vi "Increment Decrement Visibility.vi"(0 "Control in":refnum<vi>, 5 "make compliant?":bool, 11 "error in":errorcluster) -> (4 "Control out":refnum<vi>, 6 "non-compliant?":bool, 15 "error out":errorcluster)   [LabVIEW 2011, in "Align To Connector.lvlib"]
uses:
  Align To Connector.lvlib
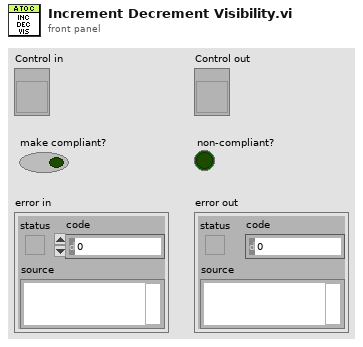
[diagram p1: front panel]
types:
  T1 = enum32{"not a typedef", "typedef", "strict typedef", "class private data"}
  T2 = typedef "LVRectTypeDef.ctl" = cluster{"Left":i16, "Top":i16, "Right":i16, "Bottom":i16}
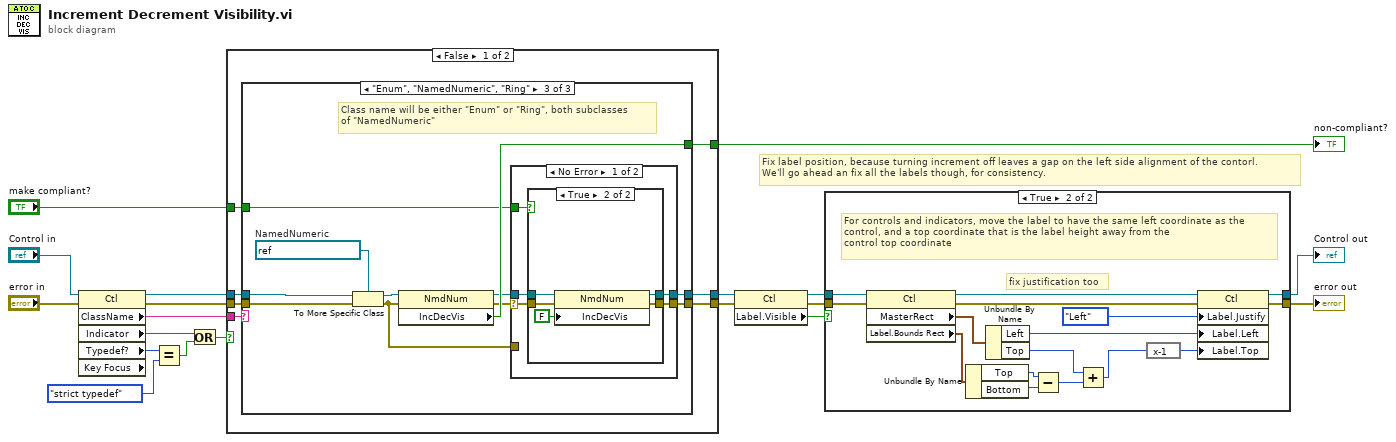
[diagram p0: block diagram]
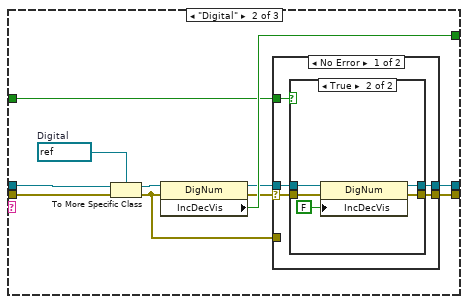
[diagram p4: hidden frame]
diagram:
  # "Fix label position, because turning increment off leaves a gap on the left side alignment of the contorl.\nWe'll go ahead an fix all the labels though, for consistency."
  n1 = property class="Ctl" props=["ClassName", "Indicator", "Typedef?", "Key Focus"](reference="Control in", error in="error in") -> (reference out=w15:refnum<vi>, error out=w14:errorcluster, "ClassName"=w8:string, "Indicator"=w13:bool, "Typedef?"=w12:T1)  [unwired: 1 out]
  n2 = Equal?(x=w12, y=T1."strict typedef" ("x")) -> (x = y?=w10:bool)
  n3 = Or(x=w13, y=w10) -> (x .or. y?=w9:bool)
  n4 = case shown="False" w9 {
    tunnel: [w26 _] -> w19
    tunnel: "make compliant?" -> [w25 _]
    tunnel: [w21 w80] -> w3
    tunnel: [w20 w79] -> w4
    tunnel: w15 -> [w24 w80]
    tunnel: w14 -> [w23 w79]
    tunnel: w8 -> [w22 _]
    frame False {
      n5 = case shown="\"Enum\", \"NamedNumeric\", \"Ring\"" w22 {
        tunnel: [_ w39 w64] -> w26
        tunnel: w25 -> [_ w30 w55]
        tunnel: [w27 w38 w57] -> w21
        tunnel: [w28 w37 w54] -> w20
        tunnel: w23 -> [w28 w34 w62]
        tunnel: w24 -> [w27 w33 w61]
        frame Default {
        }
        frame "Digital" {
          w35 = refnum<vi> refnum  # Digital
          n6 = To More Specific Class(target class=w35, reference=w33, error in=w34) -> (specific class reference=w36:refnum<vi>, error out=w29:errorcluster)
          n7 = property class="DigNum"(reference=w36, error in=w29) -> (reference out=w32:refnum<vi>, error out=w31:errorcluster, "IncDecVis"=w39:bool)
          n8 = case shown="No Error" w31 {
            selector: w31 -> [w41 _]
            tunnel: [w44 w52] -> w38
            tunnel: [w43 w53] -> w37
            tunnel: w32 -> [w42 w52]
            tunnel: w30 -> [w40 _]
            tunnel: w29 -> [_ w53]
            frame No Error {
              n9 = case shown="True" w40 {
                tunnel: [w46 w51] -> w44
                tunnel: [w45 w50] -> w43
                tunnel: w42 -> [w46 w49]
                tunnel: w41 -> [w45 w48]
                frame False {
                }
                frame True {
                  n10 = property class="DigNum"(reference=w49, error in=w48, "IncDecVis"=FALSE ("Increment/Decrement Visible?")) -> (reference out=w51:refnum<vi>, error out=w50:errorcluster)
                }
              }
            }
            frame Error {
              # "clear errors,\nsystem digital ctrls\ndon't have inc/dec"
            }
          }
        }
        frame "Enum", "NamedNumeric", "Ring" {
          w60 = refnum<vi> refnum  # NamedNumeric
          # "Class name will be either \"Enum\" or \"Ring\", both subclasses\nof \"NamedNumeric\""
          n11 = To More Specific Class(target class=w60, reference=w61, error in=w62) -> (specific class reference=w63:refnum<vi>, error out=w56:errorcluster)
          n12 = property class="NmdNum"(reference=w63, error in=w56) -> (reference out=w59:refnum<vi>, error out=w58:errorcluster, "IncDecVis"=w64:bool)
          n13 = case shown="No Error" w58 {
            selector: w58 -> [w66 _]
            tunnel: [w69 w77] -> w57
            tunnel: [w68 w78] -> w54
            tunnel: w59 -> [w67 w77]
            tunnel: w55 -> [w65 _]
            tunnel: w56 -> [_ w78]
            frame No Error {
              n14 = case shown="True" w65 {
                tunnel: [w71 w76] -> w69
                tunnel: [w70 w75] -> w68
                tunnel: w67 -> [w71 w74]
                tunnel: w66 -> [w70 w73]
                frame False {
                }
                frame True {
                  n15 = property class="NmdNum"(reference=w74, error in=w73, "IncDecVis"=FALSE ("Increment/Decrement Visible?")) -> (reference out=w76:refnum<vi>, error out=w75:errorcluster)
                }
              }
            }
            frame Error {
              # "clear errors,\nsystem digital ctrls\ndon't have inc/dec"
            }
          }
        }
      }
    }
    frame True {
      # "skip"
    }
  }
  "non-compliant?" <- w19
  n16 = property class="Ctl"(reference=w3, error in=w4) -> (reference out=w6:refnum<vi>, error out=w5:errorcluster, "Label.Visible"=w7:bool)
  n17 = case shown="True" w7 {
    tunnel: w5 -> [w82 w98]
    tunnel: w6 -> [w81 w97]
    tunnel: [w82 w96] -> w1
    tunnel: [w81 w84] -> w2
    frame False {
      # "Ignore Controls whose labels are not visible"
    }
    frame True {
      # "fix justification too"
      # "For controls and indicators, move the label to have the same left coordinate as the\ncontrol, and a top coordinate that is the label height away from the\ncontrol top coordinate"
      n18 = property class="Ctl"(reference=w97, error in=w98) -> (reference out=w90:refnum<vi>, error out=w91:errorcluster, "MasterRect"=w95:T2, "Label.Bounds Rect"=w89:T2)
      n19 = Unbundle By Name(w89) -> ("Top"=w93:i16, "Bottom"=w94:i16)
      n20 = Unbundle By Name(w95) -> ("Left"=w88:i16, "Top"=w86:i16)
      n21 = Subtract(x=w93, y=w94) -> (x-y=w92:i16)
      n22 = Add(x=w86, y=w92) -> (x+y=w87:i16)
      n23 = expression code="x-1"(w87) -> (w83:i16)
      n24 = property class="Ctl"(reference=w90, error in=w91, "Label.Justify"=enum16{"Left", "Center", "Right"}."Left" ("Label.Justification"), "Label.Left"=w88, "Label.Top"=w83) -> (reference out=w84:refnum<vi>, error out=w96:errorcluster)
    }
  }
  "Control out" <- w2
  "error out" <- w1
